vi "temp_.vi"() -> ()   [LabVIEW 2019]
uses:
  <vilib>/FPGAPlugInAG/sbRIO-9629/niLvFpga_Open_sbRIO-9629.vi
  <vilib>/rvi/interface/common/dynamic/niFpgaDynamicAddResources.vi
  <vilib>/Utility/error.llb/Error Cluster From Error Code.vi
  <vilib>/rvi/errors/niLvFpgaAdjustHostInterfaceError.vi
  <vilib>/FPGAPlugInAG/Dynamic/niLvFpga_Close_Dynamic.vi
  <vilib>/rvi/interface/nirviOpenFPGA/nirviOpenFPGA.xnode
  FPGA Bitfiles/fcmsinglesection_FPGATarget_CloseLoopMotorTu_eGt+d+EV+VE.lvbitx
  Close_Loop_Motor_Tune.vi
  <vilib>/rvi/interface/nirviReadWriteControl/nirviReadWriteControl.xnode
  <vilib>/rvi/interface/nirviCloseFPGA/nirviCloseFPGA.xnode
  NiFpgaLv.dll
  <vilib>/rvi/interface/Simulation/niFpgaSimulationCallBeginRW.vi
panel:
  out "data out":string
  out "Current Tip Position":dbl[](array[numeric])
  out "Error":dbl[](array[numeric])
  in  "Kp":dbl[](array[numeric])
  in  "Upper limit":dbl[](array[numeric])
  in  "Lower limit":dbl[](array[numeric])
  out "logical AND":bool
  out "alpha":dbl
  out "L_v":dbl
  in  "r":dbl
  in  "omega":dbl
  out "Desired Tip Position":dbl[](array[numeric])
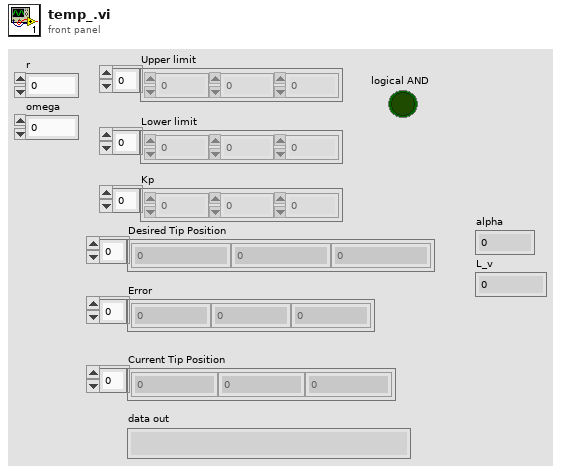
[diagram p1: front panel]
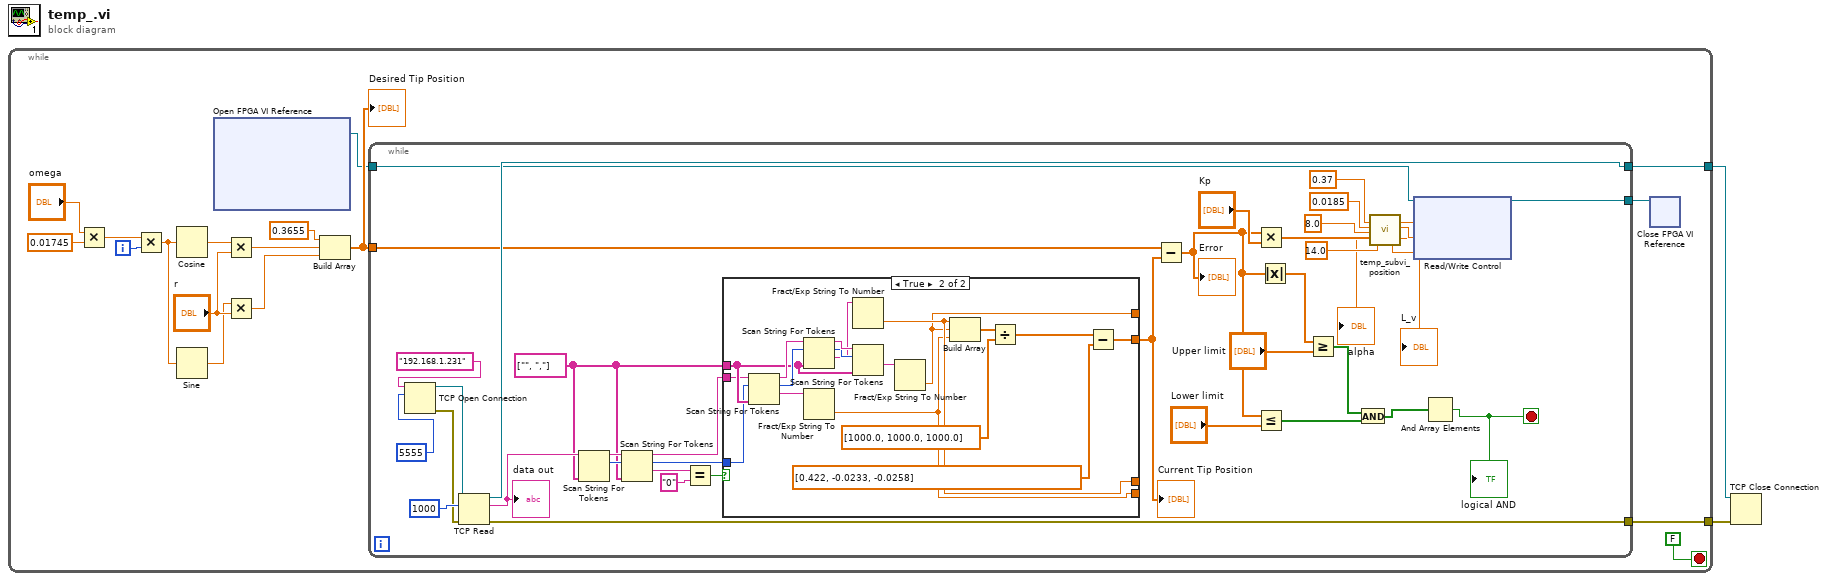
[diagram p0: block diagram]
diagram:
  n1 = while {
    tunnel: [w18] -> w2
    tunnel: [w17] -> w1
    i -> [w12]
    stop <- FALSE stop-if-true
    n2 = Multiply(x="omega", y=0.01745) -> (x*y=w13:dbl)
    n3 = Multiply(x=w13, y=w12) -> (x*y=w8:dbl)
    n4 = Cosine(x=w8) -> (cos(x)=w11:dbl)
    n5 = Sine(x=w8) -> (sin(x)=w7:dbl)
    n6 = xnode "Open FPGA VI Reference"() -> ("FPGA VI Reference Out"=w4:refnum<k20>)  [unwired: 2 in, 1 out]
    n7 = Multiply(x=w11, y="r") -> (x*y=w10:dbl)
    n8 = Multiply(x=w7, y="r") -> (x*y=w6:dbl)
    n9 = Build Array(0.3655 ("element"), w10, w6) -> (w5:dbl[])
    "Desired Tip Position" <- w5
    n10 = while {
      tunnel: [w48] -> w18
      tunnel: [w47] -> w17
      tunnel: w5 -> [w45]
      tunnel: w4 -> [w40]
      tunnel: [w39] -> w3
      stop <- w26 stop-if-true
      w51 = string[] ["", ","] ("delimiters (\\s,\\t,\\r,\\n)")
      n11 = TCP Open Connection(address="192.168.1.231", remote port or service name=u16 5555) -> (connection ID=w22:refnum<k5>, error out=w23:errorcluster)  [unwired: 3 in]
      n12 = TCP Read(connection ID=w22, bytes to read=1000, error in (no error)=w23) -> (connection ID out=w47:refnum<k5>, data out=w53:string, error out=w48:errorcluster)  [unwired: 2 in]
      "data out" <- w53
      n13 = Scan String For Tokens(6:w51, 9:w53) -> (2:w55:i32, 3:w56:string)  [unwired: 4 in, 2 out]
      n14 = Scan String For Tokens(6:w51, 8:w55, 9:w56) -> (1:w57:string, 2:w50:i32, 3:w49:string)  [unwired: 3 in, 1 out]
      n15 = Equal?(x=w57, y="0") -> (x = y?=w52:bool)
      n16 = case shown="True" w52 {
        tunnel: [_ w65] -> _
        tunnel: [_ w64] -> _
        tunnel: [_ w63] -> _
        tunnel: w51 -> [_ w62]
        tunnel: w50 -> [_ w61]
        tunnel: w49 -> [_ w60]
        tunnel: [_ w59] -> w46
        frame False {
        }
        frame True {
          n17 = Scan String For Tokens(6:w62, 8:w61, 9:w60) -> (1:w72:string, 2:w74:i32, 3:w76:string)  [unwired: 3 in, 1 out]
          n18 = Scan String For Tokens(6:w62, 8:w74, 9:w76) -> (1:w71:string, 2:w73:i32, 3:w75:string)  [unwired: 3 in, 1 out]
          n19 = Fract/Exp String To Number(string=w72) -> (number=w63:dbl)  [unwired: 3 in, 1 out]
          n20 = Fract/Exp String To Number(string=w71) -> (number=w65:dbl)  [unwired: 3 in, 1 out]
          n21 = Scan String For Tokens(6:w62, 8:w73, 9:w75) -> (1:w70:string)  [unwired: 3 in, 3 out]
          n22 = Fract/Exp String To Number(string=w70) -> (number=w64:dbl)  [unwired: 3 in, 1 out]
          n23 = Build Array(w65, w64, w63) -> (w69:dbl[])
          n24 = Divide(x=w69, y=dbl[] [1000.0, 1000.0, 1000.0]) -> (x/y=w67:dbl[])
          n25 = Subtract(x=w67, y=dbl[] [0.422, -0.0233, -0.0258]) -> (x-y=w59:dbl[])
        }
      }
      "Current Tip Position" <- w46
      n26 = Subtract(x=w45, y=w46) -> (x-y=w28:dbl[])
      "Error" <- w28
      n27 = Multiply(x=w28, y="Kp") -> (x*y=w34:dbl[])
      n28 = Less Or Equal?(x=w28, y="Lower limit") -> (x <= y?=w29:bool[])
      n29 = Absolute Value(x=w28) -> (abs(x)=w31:dbl[])
      n30 = Greater Or Equal?(x=w31, y="Upper limit") -> (x >= y?=w30:bool[])
      n31 = And(x=w30, y=w29) -> (x .and. y?=w27:bool[])
      n32 = call "temp_subvi_position.vi"("Length of the FCM (m)"=0.37, "Radius of disk (m)"=0.0185, "Number of Disks"=8.0, "Tip position"=w34, "Radius of pulley (mm)"=14.0) -> ("alpha"=→"alpha":dbl, "L_v"=→"L_v":dbl, "Theta 3"=w36:dbl, "Theta 1"=w38:dbl, "Theta 2"=w37:dbl)  [unwired: 4 in, 6 out]
      n33 = xnode "Read/Write Control"("FPGA VI Reference In"=w40, "desired angle"=w38, "desired angle 2"=w37, "desired angle 3"=w36) -> ("FPGA VI Reference Out"=w39:refnum<k20>)  [unwired: 1 in, 1 out]
      n34 = And Array Elements(Boolean array=w27) -> (logical AND=w26:bool)
      "logical AND" <- w26
    }
    n35 = xnode "Close FPGA VI Reference"("FPGA VI Reference In"=w3) -> ()  [unwired: 1 in, 1 out]
  }
  n36 = TCP Close Connection(connection ID=w1, error in (no error)=w2) -> ()  [unwired: 1 in, 2 out]
